vi "Definition.vi"(11 "Game":refnum<class "Game.lvclass">) -> (2 "Entity Definition":refnum<class "Type.lvclass">[](array[class]))   [LabVIEW 2022 SP3, in "Conditum-Example.lvlib" / "Game.lvclass"]
uses:
  Game.lvclass
  Conditum/Columns/Type/Type.lvclass
  Conditum/Columns/String/String.lvclass
  C:/dev/lv/illuminated-g/lv-conditum/Conditum/Columns/Type/Type.lvclass
  Conditum/Columns/Timestamp/Timestamp.lvclass
  Conditum/Columns/Boolean/Boolean.lvclass
  Game.lvclass/Game.ctl
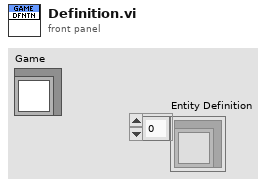
[diagram p1: front panel]
types:
  T1 = cluster{"Entity out":refnum<class "Entity.lvclass">, "Entity Collection out":refnum<class "Entity Collection.lvclass">, "String out":refnum<class "String.lvclass">, "DateTime out":refnum<class "Timestamp.lvclass">, "Boolean out":refnum<class "Boolean.lvclass">}
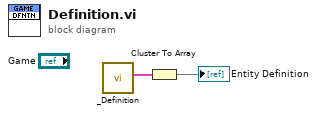
[diagram p0: block diagram]
diagram:
  n1 = call "_Definition.vi"() -> ("Definition"=w2:T1)  [unwired: 11 in]
  n2 = Cluster To Array(cluster=w2) -> (array=→"Entity Definition":refnum<class "Type.lvclass">[])
